vi "S2C_Shared_Proc_ManageEventError.vi"(8 "Error In":errorcluster) -> (0 "Error Out":errorcluster)   [LabVIEW 2024]
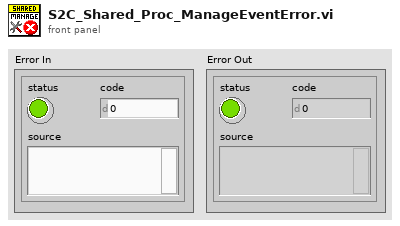
[diagram p1: front panel]
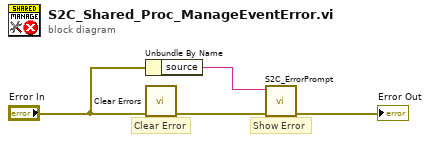
[diagram p0: block diagram]
diagram:
  # "Show Error"
  # "Clear Error"
  n1 = Unbundle By Name("Error In") -> ("source"=w2:string)
  n2 = call <vilib>:"Clear Errors.vi"("error in (no error)"="Error In") -> ("error out"=w4:errorcluster)  [unwired: 5 in, 1 out]
  n3 = call "S2C_ErrorPrompt.vi"("Error In"=w4, "ErrMsgIn"=w2) -> ("Error Out"=→"Error Out":errorcluster)  [unwired: 9 in]
